vi "BonOMM-SAOMM.Test.vi"() -> ()   [LabVIEW 2011] (continued)
                                n1894 = local read "CmdPending"() -> (w5588:bool)
                                n1895 = case shown="True" w5588 {
                                tunnel: w5589 -> [_ w5595]
                                frame False {
                                }
                                frame True {
                                n1896 = local write "Error Code"(w5595) -> ()
                                }
                                }
                                n1897 = local read "FIFO d'erreur"() -> (w5591:T7)
                                n1898 = Bundle("ETCS", w5589, w5589, "ATTENTION!!\nLa commande STOP a échoué.\nVérifiez TCS.") -> (w5592:cluster{string, i32, i32, string})  [unwired: 1 in]
                                n1899 = Build Array (concatenate)(w5591, w5592) -> (w5590:T7)
                                n1900 = local write "FIFO d'erreur"(w5590) -> ()
                                }
                                frame True {
                                }
                                }
                                }
                                }
                                }
                                }
                                }
                                }
                              }
                              frame #2 {
                                w5598 = 0
                                w5599 = 0
                                w5596 = FALSE
                                # "Voir le fonctionnement de \"CMDPENDING\""
                                n1901 = property on="ModifDome" class="Bool (strict)"("Disabled"=w5599) -> ()  [unwired: 2 in, 2 out]
                                n1902 = property on="Écran" class="Bool (strict)"("Disabled"=w5599) -> ()  [unwired: 2 in, 2 out]
                                n1903 = property on="Range" class="Bool (strict)"("Disabled"=w5599) -> ()  [unwired: 2 in, 2 out]
                                n1904 = property on="Zénith" class="Bool (strict)"("Disabled"=w5599) -> ()  [unwired: 2 in, 2 out]
                                n1905 = property on="Synctel" class="Bool (strict)"("Disabled"=w5599) -> ()  [unwired: 2 in, 2 out]
                                n1906 = property on="Offset OK" class="Bool (strict)"("Disabled"=w5599) -> ()  [unwired: 2 in, 2 out]
                                n1907 = local read "CmdPending"() -> (w5597:bool)
                                n1908 = property on="GO" class="Bool (strict)"("Disabled"=w5598) -> ()  [unwired: 2 in, 2 out]
                                n1909 = property on="ModCoor" class="Bool (strict)"("Disabled"=w5598) -> ()  [unwired: 2 in, 2 out]
                                n1910 = property on="ModifFoyer" class="Bool (strict)"("Disabled"=w5598) -> ()  [unwired: 2 in, 2 out]
                                n1911 = property on="Coupole-Tél" class="Bool (strict)"("Disabled"=w5598) -> ()  [unwired: 2 in, 2 out]
                                n1912 = case shown="True" w5597 {
                                frame False {
                                }
                                frame True {
                                n1913 = local write "CmdPending"(FALSE) -> ()
                                }
                                }
                                n1914 = local write "ModifRotation"(w5596) -> ()
                                n1915 = property on="ModifRotation" class="Bool (strict)"("Blinking"=w5596) -> ()  [unwired: 2 in, 2 out]
                              }
                            }
                          }
                        }
                      }
                    }
                    n1916 = control-ref of="TERMINAL"() -> (w5495:refnum<vi>)
                    n1917 = control-ref of="Indicateur d'état"() -> (w5494:refnum<vi>)
                    n1918 = call "TERMINAL.vi"("Indicateur Refnum"=w5494, "Terminal Refnum"=w5495, "Indicateur d'état"="Modification de la rotation de la bonnette") -> ()
                  }
                }
              }
              event "ModifFoyer": Value Change {
                n1919 = event-data() -> ()  [unwired: 1 in, 5 out]
                n1920 = case shown="True" "ModifFoyer" {
                  frame False {
                  }
                  frame True {
                    n1921 = local read "Foyer"() -> (w5602:dbl)
                    n1922 = call "Set foyer.vi"("Foyer In"=w5602) -> ("Foyer Out"=w5604:dbl, "DONE"=w5605:bool, "sortie foyer sonde"=w5603:bool)  [unwired: 1 in]
                    n1923 = case shown="True" w5605 {
                      selector: w5605 -> [w5606 _]
                      tunnel: w5604 -> [_ w5610]
                      tunnel: w5603 -> [_ w5609]
                      tunnel: w5602 -> [_ w5608]
                      frame False {
                        n1924 = local write "ModifFoyer"(w5606) -> ()
                      }
                      frame True {
                        n1925 = Bundle By Name(cluster=T22 {"newFoyer"=0.0, "updSonde"=TRUE, "oldFoyer"=0.0}, "newFoyer"=w5610, "updSonde"=w5609, "oldFoyer"=w5608) -> (w5607:T22)
                        n1926 = call "EnqueueEvents.vi"("data"=w5607, "message"="Foyer.Ajuster") -> ()  [unwired: 1 in]
                      }
                    }
                  }
                }
              }
              event "ModifDome": Value Change {
                n1927 = event-data() -> ("NewVal"=w5613:bool)  [unwired: 1 in, 4 out]
                n1928 = case shown="True" w5613 {
                  frame False {
                  }
                  frame True {
                    n1929 = local read "Coupole"() -> (w5614:dbl)
                    n1930 = Number To Decimal String(number=w5614) -> (decimal integer string=w5615:string)  [unwired: 1 in]
                    n1931 = call "Set dome.vi"("Dome In"=w5614) -> ("DONE"=w5621:bool, "Dome Out"=w5620:dbl)
                    n1932 = Concatenate Strings("Synchronisation de la coupole sur " ("string"), w5615) -> (w5617:string)
                    n1933 = case shown="True" w5621 {
                      selector: w5621 -> [w5622 _]
                      tunnel: w5620 -> [_ w5623]
                      frame False {
                        n1934 = local write "ModifDome"(w5622) -> ()
                      }
                      frame True {
                        n1935 = stacked-sequence {
                          tunnel: w5623 -> [_ w5633 _]
                          frame #0 {
                            n1936 = control-ref of="TCS C actif"() -> (w5624:refnum<vi>)
                            n1937 = call "TCS-Wait4Flag.vi"("Raise Flag ?"=TRUE, "Ctl Refnum IN"=w5624) -> ()  [unwired: 8 in, 2 out]
                          }
                          frame #1 {
                            n1938 = control-ref of="TCS actif"() -> (w5626:refnum<vi>)
                            n1939 = local read "TCS VRN"() -> (w5632:refnum<visa-resource-name>)
                            n1940 = Build Array(w5633) -> (w5629:dbl[])
                            n1941 = call "EXCOM-CMD.vi"("VRN IN"=w5632, "Bool Refnum"=w5626, "Commande #"=2 ("NombredArguments"), "Args"=w5629) -> ("VRN OUT"=w5630:refnum<visa-resource-name>, "OK Done"=w5628:bool, "Error OUT"=w5627:errorcluster)  [unwired: 9 in]
                            n1942 = local write "TCS VRN"(w5630) -> ()
                            n1943 = local write "TCS Error"(w5627) -> ()
                            n1944 = case shown="False" w5628 {
                              selector: w5628 -> [w5634 w5638]
                              frame False {
                                n1945 = local write "ModifDome"(w5634) -> ()
                                n1946 = One Button Dialog(message="ATTENTION!!\nProblème d'ajustement\nde la position de la coupole.\nVérifiez TCS.", button name ("OK")="OK" ("nom du bouton (\"OK\")")) -> ()  [unwired: 1 out]
                              }
                              frame True {
                                n1947 = Not(x=w5638) -> (.not. x?=w5637:bool)
                                n1948 = local write "ModifDome"(w5637) -> ()
                              }
                            }
                          }
                          frame #2 {
                            n1949 = local write "TCS actif"(FALSE ("BONC-TCS")) -> ()
                          }
                        }
                      }
                    }
                    n1950 = control-ref of="TERMINAL"() -> (w5619:refnum<vi>)
                    n1951 = control-ref of="Indicateur d'état"() -> (w5618:refnum<vi>)
                    n1952 = call "TERMINAL.vi"("Indicateur Refnum"=w5618, "Terminal Refnum"=w5619, "Indicateur d'état"=w5617) -> ()
                  }
                }
              }
              event "Coupole-Tél": Value Change {
                n1953 = event-data() -> ()  [unwired: 1 in, 5 out]
                n1954 = Select(t="ON" ("string"), s="Coupole-Tél", f="OFF" ("string")) -> (s? t:f=w5649:string)
                n1955 = control-ref of="TERMINAL"() -> (w5653:refnum<vi>)
                n1956 = control-ref of="Indicateur d'état"() -> (w5652:refnum<vi>)
                n1957 = Concatenate Strings("AUTO DOME : " ("string"), w5649) -> (w5650:string)
                n1958 = call "TERMINAL.vi"("Indicateur Refnum"=w5652, "Terminal Refnum"=w5653, "Indicateur d'état"=w5650) -> ()
                n1959 = Boolean To (0,1)(Boolean="Coupole-Tél") -> (0, 1=w5655:i16)
                n1960 = To Double Precision Float(number=w5655) -> (double precision float=w5645:dbl)
                n1961 = Build Array(w5645) -> (w5644:dbl[])
                n1962 = control-ref of="TCS actif"() -> (w5640:refnum<vi>)
                n1963 = local read "TCS VRN"() -> (w5654:refnum<visa-resource-name>)
                n1964 = call "EXCOM-CMD.vi"("VRN IN"=w5654, "Bool Refnum"=w5640, "Commande #"=20 ("NombredArguments"), "Args"=w5644) -> ("VRN OUT"=w5643:refnum<visa-resource-name>, "OK Done"=w5641:bool, "Error OUT"=w5642:errorcluster)  [unwired: 9 in]
                n1965 = local write "TCS Error"(w5642) -> ()
                n1966 = local write "TCS VRN"(w5643) -> ()
                n1967 = case shown="False" w5641 {
                  frame False {
                    n1968 = One Button Dialog(message="ATTENTION!!\nLa commande DOME ON/OFF a échoué.\nVérifiez TCS.", button name ("OK")="OK" ("nom du bouton (\"OK\")")) -> ()  [unwired: 1 out]
                  }
                  frame True {
                  }
                }
              }
              event "Offset OK": Value Change {
                n1969 = event-data() -> ("NewVal"=w5659:bool)  [unwired: 1 in, 4 out]
                n1970 = case shown="True" w5659 {
                  frame False {
                  }
                  frame True {
                    # "OFFSET en\nsecondes d'arc"
                    # "Commande OFFSET\nSlew Enable"
                    # "MX"
                    # "MY"
                    # "Y"
                    # "X"
                    # "DEC"
                    # "AD"
                    n1971 = stacked-sequence {
                      seq-local: [_ w5704 _] -> [_ _ w5725]
                      tunnel: "Offset DEC" -> [w5668 w5702 _]
                      tunnel: "Offset RA" -> [w5671 w5703 _]
                      frame #0 {
                        n1972 = Number To Fractional String(number=w5668, precision (6)=i16 2) -> (F-format string=w5664:string)  [unwired: 2 in]
                        n1973 = Number To Fractional String(number=w5671, precision (6)=i16 2) -> (F-format string=w5666:string)  [unwired: 2 in]
                        n1974 = Concatenate Strings("Envoi manuel d'un offset de " ("string"), w5666, ", " ("string"), w5664) -> (w5663:string)
                        n1975 = local write "Offset OK"(FALSE) -> ()
                        n1976 = control-ref of="TERMINAL"() -> (w5672:refnum<vi>)
                        n1977 = control-ref of="Indicateur d'état"() -> (w5673:refnum<vi>)
                        n1978 = call "TERMINAL.vi"("Indicateur Refnum"=w5673, "Terminal Refnum"=w5672, "Indicateur d'état"=w5663) -> ()
                        "Offset en cours" <- TRUE ("Offset en cours")
                      }
                      frame #1 {
                        n1979 = control-ref of="MovingXY"() -> (w5676:refnum<vi>)
                        n1980 = control-ref of="SNR"() -> (w5677:refnum<vi>)
                        n1981 = control-ref of="TCS actif"() -> (w5697:refnum<vi>)
                        n1982 = control-ref of="Table actif"() -> (w5696:refnum<vi>)
                        n1983 = control-ref of="Position Z"() -> (w5695:refnum<vi>)
                        n1984 = control-ref of="StartServo"() -> (w5694:refnum<vi>)
                        n1985 = control-ref of="Mode"() -> (w5689:refnum<vi>)
                        n1986 = control-ref of="Servo"() -> (w5693:refnum<vi>)
                        n1987 = control-ref of="StopServo"() -> (w5692:refnum<vi>)
                        n1988 = control-ref of="DiffX"() -> (w5690:refnum<vi>)
                        n1989 = control-ref of="DiffY"() -> (w5691:refnum<vi>)
                        n1990 = local read "TableAstrom"() -> (w5686:T4)
                        n1991 = local read "FieldAstrom"() -> (w5688:T4)
                        n1992 = local read "GuiderAstrom"() -> (w5687:T4)
                        n1993 = local read "TCS VRN"() -> (w5685:refnum<visa-resource-name>)
                        n1994 = local read "TCS Error"() -> (w5684:errorcluster)
                        n1995 = local read "Table VRN"() -> (w5683:refnum<visa-resource-name>)
                        n1996 = local read "Table Error"() -> (w5682:errorcluster)
                        n1997 = Bundle("TableAstrom"=w5686, "FieldAstrom"=w5688, "GuiderAstrom"=w5687) -> (w5680:T40)  [unwired: 1 in]
                        n1998 = Bundle("TCS VRN"=w5685, "TCS Error"=w5684, "Table VRN"=w5683, "Table Error"=w5682) -> (w5679:T41)  [unwired: 1 in]
                        n1999 = Bundle("TCS actif"=w5697, "Table actif"=w5696, "Position Z"=w5695, "StartServo"=w5694, "Mode"=w5689, "Servo"=w5693, "StopServo"=w5692, "DiffX"=w5690, "DiffY"=w5691, "SNR"=w5677, "MovingXY"=w5676) -> (w5681:T42)  [unwired: 1 in]
                        n2000 = local read "OffsetAcc"() -> (w5678:dbl)
                        n2001 = while {
                          tunnel: [FALSE] -> w5675
                          stop <- w5707 continue-if-true
                          n2002 = local read "enfoncé"() -> (w5709:bool)
                          n2003 = Wait (ms)(milliseconds to wait=u32 200) -> ()  [unwired: 1 out]
                          n2004 = Not(x=w5709) -> (.not. x?=w5708:bool)
                          n2005 = local write "enfoncé"(w5708) -> ()
                          n2006 = local read "Offset en cours"() -> (w5707:bool)
                        }
                        n2007 = call "Cheesy_Offset.vi"("Communications_Cluster"=w5679, "Astrom_Cluster"=w5680, "RA offset"=w5703, "DEC offset"=w5702, "VariablesReferences"=w5681, "OffsetAccuracy (pixels)"=w5678) -> ("Error code"=w5701:u8, "Undo offset"=w5704:bool, "Warning code"=w5700:u8)  [unwired: 6 in, 1 out]
                        n2008 = To Unsigned Long Integer(number=w5700) -> (unsigned 32bit integer=w5698:u32)
                        n2009 = To Unsigned Long Integer(number=w5701) -> (unsigned 32bit integer=w5699:u32)
                        n2010 = flat-sequence {
                          tunnel: w5699 -> [w5713]
                          tunnel: w5698 -> [w5712]
                          frame #0 {
                            w5714 = u32 0 ("Error Code IN")
                            n2011 = local read "FIFO d'erreur"() -> (w5711:T7)
                            n2012 = call "Error_Format.vi"("FIFO IN"=w5711, "Error Code IN"=w5714, "Warning Code IN"=w5714, "Error Bit"=w5713, "Warning Bit"=w5712, "Source"="offset") -> ("FIFO OUT"=w5710:T7)  [unwired: 11 in, 2 out]
                            n2013 = local write "FIFO d'erreur"(w5710) -> ()
                          }
                          frame #1 {
                            n2014 = local write "Offset en cours"(FALSE ("Offset en cours")) -> ()
                          }
                        }
                        n2015 = local write "enfoncé"(w5675) -> ()
                      }
                      frame #2 {
                        w5726 = FALSE
                        # "Utile ?"
                        n2016 = local read "Table VRN"() -> (w5719:refnum<visa-resource-name>)
                        n2017 = local read "Table Error"() -> (w5718:errorcluster)
                        n2018 = control-ref of="Table actif"() -> (w5717:refnum<vi>)
                        n2019 = call "Newmark-Stop.vi"("Table VRN IN"=w5719, "Bool Refnum"=w5717, "Error IN"=w5718) -> ("Table VRN OUT"=w5721:refnum<visa-resource-name>, "Error OUT"=w5720:errorcluster)  [unwired: 11 in]
                        n2020 = local write "Table Error"(w5720) -> ()
                        n2021 = local write "Table VRN"(w5721) -> ()
                        n2022 = local write "RangeTable"(w5726) -> ()
                        n2023 = local write "Calibration"(w5726) -> ()
                        n2024 = local write "stoptable"(w5726) -> ()
                        n2025 = local write "Alacible"(w5726) -> ()
                        n2026 = local write "Origine"(w5726) -> ()
                        n2027 = local write "Centre"(w5726) -> ()
                        n2028 = case shown="False" w5725 {
                          tunnel: [" : réussi" " : échoué"] -> w5723
                          frame False {
                          }
                          frame True {
                          }
                        }
                        n2029 = local read "TERMINAL"() -> (w5724:string)
                        n2030 = Concatenate Strings(w5724, w5723) -> (w5722:string)
                        n2031 = local write "TERMINAL"(w5722) -> ()
                      }
                    }
                  }
                }
              }
              event "ChoixFiltre": Value Change {
                n2032 = event-data() -> ()  [unwired: 1 in, 5 out]
                n2033 = local read "MC-BonOMM VRN"() -> (w5729:refnum<visa-resource-name>)
                n2034 = stacked-sequence {
                  seq-local: [w5737 _ _ _] -> [_ w5800 _ _]
                  seq-local: [w5745 _ _ _] -> [_ w5797 _ _]
                  tunnel: w5729 -> [_ w5799 _ w5846]
                  frame #0 {
                    w5749 = 2
                    n2035 = local read "F#"() -> (w5735:i32)
                    n2036 = Number To Decimal String(number=w5735) -> (decimal integer string=w5736:string)  [unwired: 1 in]
                    n2037 = control-ref of="TERMINAL"() -> (w5741:refnum<vi>)
                    n2038 = control-ref of="Indicateur d'état"() -> (w5742:refnum<vi>)
                    n2039 = Unbundle("ChoixFiltre") -> ("filtre #1"=w5752:bool, "filtre #2"=w5753:bool, "filtre #3"=w5754:bool, "filtre #4"=w5755:bool, "filtre #5"=w5756:bool, "filtre #6"=w5757:bool)
                    n2040 = Build Array(w5752, w5753, w5754, w5755, w5756, w5757) -> (w5758:bool[])
                    n2041 = Search 1D Array(1D array=w5758, element=TRUE) -> (index of element=w5743:i32)  [unwired: 1 in]
                    n2042 = Increment(x=w5743) -> (x+1=w5737:i32)
                    n2043 = Number To Decimal String(number=w5737) -> (decimal integer string=w5738:string)  [unwired: 1 in]
                    n2044 = Concatenate Strings("Passage du filtre #", w5736, " au filtre #", w5738) -> (w5734:string)
                    n2045 = call "TERMINAL.vi"("Indicateur Refnum"=w5742, "Terminal Refnum"=w5741, "Indicateur d'état"=w5734) -> ()
                    n2046 = Not Equal To 0?(x=w5737) -> (x != 0?=w5744:bool)
                    n2047 = property on="ChoixFiltre" class="Clust (strict)"() -> ("Controls[]"=w5748:refnum<vi>[])  [unwired: 2 in, 2 out]
                    n2048 = case shown="True" w5744 {
                      selector: w5744 -> [w5782 _]
                      tunnel: w5743 -> [_ w5785]
                      tunnel: [w5782 w5784] -> w5745
                      frame False {
                      }
                      frame True {
                        n2049 = local read "Bypass Tech"() -> (w5783:bool)
                        n2050 = case shown="True" w5783 {
                          selector: w5783 -> [_ w5795]
                          tunnel: w5785 -> [w5793 _]
                          tunnel: [w5786 w5795] -> w5784
                          frame False {
                            n2051 = local read "Tableau des filtres"() -> (w5794:string[])
                            n2052 = Index Array(array=w5794, index=w5793) -> (element=w5792:string)
                            n2053 = Concatenate Strings("Désirez-vous passer au filtre " ("message"), w5792, " ?" ("message")) -> (w5789:string)
                            n2054 = Two Button Dialog(message=w5789, 1:"NON" ("F button name (\"Cancel\")"), 2:"OUI" ("T button name (\"OK\")")) -> (T button?=w5786:bool)
                          }
                          frame True {
                          }
                        }
                      }
                    }
                    n2055 = Index Array(array=w5748, index=w5743) -> (element=w5747:refnum<vi>)
                    n2056 = property class="Ctl"(reference=w5747, "Blinking"=TRUE) -> ()  [unwired: 1 in, 2 out]
                    n2057 = Index Array(array=w5748, index #1=0 ("indice"), index #2=1 ("indice"), index #3=2 ("indice"), index #4=3 ("indice"), index #5=4 ("indice"), index #6=5 ("indice")) -> (element #1=w5760:refnum<vi>, element #2=w5761:refnum<vi>, element #3=w5762:refnum<vi>, element #4=w5763:refnum<vi>, element #5=w5764:refnum<vi>, element #6=w5765:refnum<vi>)
                    n2058 = property class="Ctl"(reference=w5760, "Disabled"=w5749) -> ()  [unwired: 1 in, 2 out]
                    n2059 = property class="Ctl"(reference=w5761, "Disabled"=w5749) -> ()  [unwired: 1 in, 2 out]
                    n2060 = property class="Ctl"(reference=w5762, "Disabled"=w5749) -> ()  [unwired: 1 in, 2 out]
                    n2061 = property class="Ctl"(reference=w5763, "Disabled"=w5749) -> ()  [unwired: 1 in, 2 out]
                    n2062 = property class="Ctl"(reference=w5764, "Disabled"=w5749) -> ()  [unwired: 1 in, 2 out]
                    n2063 = property class="Ctl"(reference=w5765, "Disabled"=w5749) -> ()  [unwired: 1 in, 2 out]
                    n2064 = local read "Tableau des filtres"() -> (w5733:string[])
                    n2065 = Current VI's Menubar() -> (w5730:refnum<k9>)
                    n2066 = for {
                      tunnel: w5733 -> [w5774] mode=indexing
                      tunnel: "@@" -> [w5778]
                      tunnel: "raf_" -> [w5779]
                      tunnel: w5730 -> [w5775]
                      tunnel: [w5773] -> _ mode=indexing
                      i -> [w5780]
                      n2067 = Number To Decimal String(number=w5780, width (-)=i16 1) -> (decimal integer string=w5777:string)
                      n2068 = Concatenate Strings(w5779, w5774, w5778, w5777) -> (w5776:string)
                      n2069 = Set Menu Item Info(6:FALSE ("checked"), 7:w5776, 9:TRUE ("enabled"), 10:w5774, 11:w5775) -> (0:w5773:errorcluster)  [unwired: 2 in, 1 out]
                    }
                  }
                  frame #1 {
                    n2070 = Not Equal To 0?(x=w5800) -> (x != 0?=w5798:bool)
                    n2071 = And(x=w5798, y=w5797) -> (x .and. y?=w5796:bool)
                    n2072 = case shown="True" w5796 {
                      tunnel: w5800 -> [_ w5801]
                      tunnel: w5799 -> [_ w5802]
                      frame False {
                      }
                      frame True {
                        n2073 = Number To Decimal String(number=w5801, width (-)=i16 1) -> (decimal integer string=w5803:string)
                        n2074 = VISA Write(VISA resource name=w5802, write buffer=w5803) -> (VISA resource name out=w5804:refnum<visa-resource-name>)  [unwired: 1 in, 2 out]
                        n2075 = while {
                          tunnel: w5804 -> [w5814]
                          tunnel: w5801 -> [w5813]
                          stop <- w5812 stop-if-true
                          n2076 = while {
                            tunnel: w5814 -> [w5825]
                            tunnel: [w5824] -> w5809
                            tunnel: [w5823] -> w5807
                            i -> [w5828]
                            stop <- w5821 stop-if-true
                            n2077 = local read "Annulation en cours"() -> (w5820:bool)
                            n2078 = property class="Instr"(reference=w5825) -> (reference out=w5824:refnum<visa-resource-name>, "Serial Settings:Number of Bytes at Serial Port"=w5829:u32)  [unwired: 1 in, 1 out]
                            n2079 = Not Equal To 0?(x=w5829) -> (x != 0?=w5823:bool)
                            n2080 = call "Max-iteration.vi"("i max"=100, "i act"=w5828, "Valeur entrante"=w5823) -> ("break ?"=w5822:bool)
                            n2081 = Or(x=w5820, y=w5822) -> (x .or. y?=w5821:bool)
                            n2082 = Wait Until Next ms Multiple(millisecond multiple=u32 100) -> ()  [unwired: 1 out]
                          }
                          n2083 = case shown="True" w5807 {
                            tunnel: w5809 -> [_ w5819]
                            tunnel: [0 w5816] -> w5808
                            frame False {
                            }
                            frame True {
                              n2084 = VISA Read(VISA resource name=w5819, byte count=u32 1) -> (read buffer=w5817:string)  [unwired: 1 in, 3 out]
                              n2085 = Decimal String To Number(string=w5817) -> (number=w5816:i32)  [unwired: 2 in, 1 out]
                            }
                          }
                          n2086 = Not(x=w5807) -> (.not. x?=w5811:bool)
                          n2087 = local write "F#"(w5808) -> ()
                          n2088 = Equal?(x=w5808, y=w5813) -> (x = y?=w5806:bool)
                          n2089 = local read "Annulation en cours"() -> (w5810:bool)
                          n2090 = Compound Arithmetic op=OR(w5806, w5811, w5810) -> (w5812:bool)
                        }
                      }
                    }
                  }
                  frame #2 {
                    n2091 = local read "Annulation en cours"() -> (w5830:bool)
                    n2092 = case shown="False" w5830 {
                      frame False {
                        n2093 = local read "MC_connect"() -> (w5831:bool)
                        n2094 = Wait (ms)(milliseconds to wait=u32 500) -> ()  [unwired: 1 out]
                        n2095 = case shown="False" w5831 {
                          frame False {
                            n2096 = One Button Dialog(message="Errreur lors du déplacement de la roue") -> ()  [unwired: 1 in, 1 out]
                          }
                          frame True {
                          }
                        }
                      }
                      frame True {
                      }
                    }
                  }
                  frame #3 {
                    w5837 = u8 0 ("byte count")
                    w5847 = FALSE
                    n2097 = local read "Annulation en cours"() -> (w5834:bool)
                    n2098 = case shown="False" w5834 {
                      tunnel: w5846 -> [w5869 _]
                      frame False {
                        n2099 = call "MC-BonOMM_talker.vi"("MC-BonOMM VRN"=w5869, "Commande"="q" ("write buffer"), "byte count"=u32 1, "Timeout (ms)"=1000, "answer=command?"=FALSE) -> ("Answer"=w5864:string, "ok ?"=w5863:bool)
                        n2100 = local write "MC_connect"(w5863) -> ()
                        n2101 = Decimal String To Number(string=w5864) -> (number=w5868:i32)  [unwired: 2 in, 1 out]
                        n2102 = local write "F#"(w5868) -> ()
                        n2103 = case shown="1..6" w5868 {
                          selector: w5868 -> [w5879 _]
                          frame 1..6 {
                            w5870 = TRUE ("enabled")
                            n2104 = Decrement(x=w5879) -> (x-1=w5871:i32)
                            n2105 = local read "Tableau des filtres"() -> (w5880:string[])
                            n2106 = Index Array(array=w5880, index=w5871) -> (element=w5872:string)
                            n2107 = Number To Decimal String(number=w5871, width (-)=i16 1) -> (decimal integer string=w5876:string)
                            n2108 = local write "filtre_nom"(w5872) -> ()
                            n2109 = Concatenate Strings("raf_", w5872, "@@", w5876) -> (w5878:string)
                            n2110 = Current VI's Menubar() -> (w5877:refnum<k9>)
                            n2111 = Set Menu Item Info(6:w5870, 7:w5878, 9:w5870, 10:w5872, 11:w5877) -> ()  [unwired: 2 in, 2 out]
                          }
                          frame 0, Default {
                            n2112 = local write "filtre_nom"("") -> ()
                          }
                        }
                      }
                      frame True {
                        n2113 = local read "MC-BonOMM VRN"() -> (w5883:refnum<visa-resource-name>)
                        n2114 = local read "Périphérique"() -> (w5887:u16)
                        n2115 = VISA Write(VISA resource name=w5883, write buffer="r") -> (VISA resource name out=w5884:refnum<visa-resource-name>)  [unwired: 1 in, 2 out]
                        n2116 = Equal To 0?(x=w5887) -> (x = 0?=w5888:bool)
                        n2117 = Select(t="f", s=w5888, f="o") -> (s? t:f=w5891:string)
                        n2118 = flat-sequence {
                          tunnel: w5884 -> [w5913]
                          tunnel: [w5913] -> w5894
                          frame #0 {
                            n2119 = Wait (ms)(milliseconds to wait=u32 2000) -> ()  [unwired: 1 out]
                          }
                        }
                        n2120 = call "MC-BonOMM_talker.vi"("MC-BonOMM VRN"=w5894, "Commande"=w5891, "byte count"=u32 1, "Timeout (ms)"=2000, "answer=command?"=TRUE) -> ("ok ?"=w5882:bool)  [unwired: 1 out]
                        n2121 = local write "MC_connect"(w5882) -> ()
                        n2122 = case shown="True" w5882 {
                          tunnel: w5894 -> [_ w5896]
                          frame False {
                            n2123 = One Button Dialog(message="Erreur lors de l'arrêt, essayez \"reconnecter\"") -> ()  [unwired: 1 in, 1 out]
                          }
                          frame True {
                            n2124 = flat-sequence {
                              tunnel: [w5906] -> w5897
                              tunnel: w5896 -> [w5905]
                              frame #0 {
                                n2125 = Wait (ms)(milliseconds to wait=u32 500) -> ()  [unwired: 1 out]
                              }
                              frame #1 {
                                n2126 = call "MC-BonOMM_talker.vi"("MC-BonOMM VRN"=w5905, "Commande"="q", "byte count"=u32 1, "Timeout (ms)"=8000, "answer=command?"=FALSE) -> ("Answer"=w5901:string, "ok ?"=w5900:bool)
                                n2127 = local write "MC_connect"(w5900) -> ()
                                n2128 = Decimal String To Number(string=w5901) -> (number=w5906:i32)  [unwired: 2 in, 1 out]
                              }
                            }
                            n2129 = local write "F#"(w5897) -> ()
                            n2130 = case shown="1..6" w5897 {
                              selector: w5897 -> [w5907 _]
                              frame 1..6 {
                                n2131 = Decrement(x=w5907) -> (x-1=w5910:i32)
                                n2132 = local read "Tableau des filtres"() -> (w5908:string[])
                                n2133 = Index Array(array=w5908, index=w5910) -> (element=w5909:string)
                                n2134 = local write "filtre_nom"(w5909) -> ()
                              }
                              frame 0, Default {
                                n2135 = local write "filtre_nom"("") -> ()
                              }
                            }
                          }
                        }
                      }
                    }
                    n2136 = property on="ChoixFiltre" class="Clust (strict)"() -> ("Controls[]"=w5848:refnum<vi>[])  [unwired: 2 in, 2 out]
                    n2137 = Index Array(array=w5848, index #1=0 ("indice"), index #2=1 ("indice"), index #3=2 ("indice"), index #4=3 ("indice"), index #5=4 ("indice"), index #6=5 ("indice")) -> (element #1=w5850:refnum<vi>, element #2=w5851:refnum<vi>, element #3=w5852:refnum<vi>, element #4=w5853:refnum<vi>, element #5=w5854:refnum<vi>, element #6=w5855:refnum<vi>)
                    n2138 = property class="Ctl"(reference=w5850, "Blinking"=w5847) -> (reference out=w5845:refnum<vi>)  [unwired: 1 in, 1 out]
                    n2139 = property class="Ctl"(reference=w5851, "Blinking"=w5847) -> (reference out=w5844:refnum<vi>)  [unwired: 1 in, 1 out]
                    n2140 = property class="Ctl"(reference=w5852, "Blinking"=w5847) -> (reference out=w5843:refnum<vi>)  [unwired: 1 in, 1 out]
                    n2141 = property class="Ctl"(reference=w5853, "Blinking"=w5847) -> (reference out=w5842:refnum<vi>)  [unwired: 1 in, 1 out]
                    n2142 = property class="Ctl"(reference=w5854, "Blinking"=w5847) -> (reference out=w5841:refnum<vi>)  [unwired: 1 in, 1 out]
                    n2143 = property class="Ctl"(reference=w5855, "Blinking"=w5847) -> (reference out=w5840:refnum<vi>)  [unwired: 1 in, 1 out]
                    n2144 = Bundle(w5847, w5847, w5847, w5847, w5847, w5847) -> (w5861:cluster{bool, bool, bool, bool, bool, bool})  [unwired: 1 in]
                    n2145 = local read "Périphérique"() -> (w5839:u16)
                    n2146 = property class="Ctl"(reference=w5845, "Disabled"=w5837) -> ()  [unwired: 1 in, 2 out]
                    n2147 = property class="Ctl"(reference=w5844, "Disabled"=w5837) -> ()  [unwired: 1 in, 2 out]
                    n2148 = property class="Ctl"(reference=w5843, "Disabled"=w5837) -> ()  [unwired: 1 in, 2 out]
                    n2149 = property class="Ctl"(reference=w5842, "Disabled"=w5837) -> ()  [unwired: 1 in, 2 out]
                    n2150 = property class="Ctl"(reference=w5841, "Disabled"=w5837) -> ()  [unwired: 1 in, 2 out]
                    n2151 = property on="ChoixFiltre" class="Clust (strict)"("Value"=w5861) -> ()  [unwired: 2 in, 2 out]
                    n2152 = Equal To 0?(x=w5839) -> (x = 0?=w5838:bool)
                    n2153 = Select(t=w5837, s=w5838, f=u8 2) -> (s? t:f=w5835:u8)
                    n2154 = property class="Ctl"(reference=w5840, "Disabled"=w5835) -> ()  [unwired: 1 in, 2 out]
                  }
                }
              }
              event "Périphérique", "reconnect": Value Change {
                n2155 = event-data() -> ()  [unwired: 1 in, 5 out]
                n2156 = Equal?(x="Périphérique", y=u16 3) -> (x = y?=w5934:bool)
                n2157 = Equal?(x="Périphérique", y=u16 4) -> (x = y?=w5937:bool)
                n2158 = property on="AngOK" class="Bool"("Visible"=w5937) -> ()  [unwired: 2 in, 2 out]
                n2159 = property on="PAS" class="DigNum (strict)"("Visible"=w5937) -> ()  [unwired: 2 in, 2 out]
                n2160 = property on="ANG+" class="Bool"("Visible"=w5937) -> ()  [unwired: 2 in, 2 out]
                n2161 = property on="Set angle" class="DigNum (strict)"("Visible"=w5937) -> ()  [unwired: 2 in, 2 out]
                n2162 = property on="ANG-" class="Bool"("Visible"=w5937) -> ()  [unwired: 2 in, 2 out]
                n2163 = property on="Arc" class="Bool (strict)"("Visible"=w5934) -> ()  [unwired: 2 in, 2 out]
                n2164 = property on="Flat" class="Bool (strict)"("Visible"=w5934) -> ()  [unwired: 2 in, 2 out]
                n2165 = property on="Néon" class="Bool (strict)"("Visible"=w5934) -> ()  [unwired: 2 in, 2 out]
                n2166 = Equal?(x="Périphérique", y=u16 2) -> (x = y?=w5925:bool)
                n2167 = local write "reconnect"(FALSE ("reconnect")) -> ()
                n2168 = property on="SET ZERO" class="Bool"("Visible"=w5925) -> ()  [unwired: 2 in, 2 out]
                n2169 = property on="ST+" class="Bool (strict)"("Visible"=w5925) -> ()  [unwired: 2 in, 2 out]
                n2170 = property on="ST-" class="Bool (strict)"("Visible"=w5925) -> ()  [unwired: 2 in, 2 out]
                n2171 = property on="ST_RAZ" class="Bool"("Visible"=w5925) -> ()  [unwired: 2 in, 2 out]
                n2172 = property on="ST_SPD" class="Slide (strict)"("Visible"=w5925) -> ()  [unwired: 2 in, 2 out]
                n2173 = Equal?(x="Périphérique", y=u16 0) -> (x = y?=w5927:bool)
                n2174 = Equal?(x="Périphérique", y=u16 1) -> (x = y?=w5926:bool)
                n2175 = Or(x=w5927, y=w5926) -> (x .or. y?=w5915:bool)
                n2176 = Select(t=u8 0 ("y"), s=w5927, f=u8 2 ("y")) -> (s? t:f=w5930:u8)
                n2177 = property on="filtre #6" class="Bool (strict)"("Disabled"=w5930) -> ()  [unwired: 2 in, 2 out]
                n2178 = Build Array(w5927, w5926, w5925) -> (w5924:bool[])
                n2179 = Or(x=w5915, y=w5925) -> (x .or. y?=w5916:bool)
                n2180 = property on="reconnect" class="Bool (strict)"("Visible"=w5916) -> ()  [unwired: 2 in, 2 out]
                n2181 = Boolean Array To Number(Boolean array=w5924) -> (number=w5923:u32)
                n2182 = property on="ChoixFiltre" class="Clust (strict)"("Visible"=w5915) -> ()  [unwired: 2 in, 2 out]
                n2183 = property on="filtre_nom" class="Str"("Visible"=w5915) -> ()  [unwired: 2 in, 2 out]
                n2184 = property on="q-raf" class="Bool (strict)"("Visible"=w5915) -> ()  [unwired: 2 in, 2 out]
                n2185 = property on="cancel-raf" class="Bool (strict)"("Visible"=w5915) -> ()  [unwired: 2 in, 2 out]
                n2186 = property on="change_filtre_liste" class="Bool (strict)"("Visible"=w5915) -> ()  [unwired: 2 in, 2 out]
                n2187 = property on="F#" class="DigNum (strict)"("Visible"=w5915) -> ()  [unwired: 2 in, 2 out]
                n2188 = case shown="True" w5916 {
                  tunnel: w5923 -> [_ w5940]
                  frame False {
                  }
                  frame True {
                    n2189 = flat-sequence {
                      tunnel: w5940 -> [w5944]
                      tunnel: [w5944] -> w5939
                      tunnel: w5939 -> [w5964]
                      frame #0 {
                        n2190 = flat-sequence {
                          tunnel: w5941 -> [w5948]
                          frame #0 {
                            n2191 = Wait (ms)(milliseconds to wait=u32 2000) -> ()  [unwired: 1 out]
                          }
                          frame #1 {
                            n2192 = property class="Instr"(reference=w5948) -> (reference out=w5947:refnum<visa-resource-name>, "Serial Settings:Number of Bytes at Serial Port"=w5946:u32)  [unwired: 1 in, 1 out]
                            n2193 = local write "MC_connect"(FALSE ("MC_connect")) -> ()
                            n2194 = VISA Read(VISA resource name=w5947, byte count=w5946) -> ()  [unwired: 1 in, 4 out]
                          }
                        }
                        n2195 = local read "MC-BonOMM VRN"() -> (w5943:refnum<visa-resource-name>)
                        n2196 = VISA Write(VISA resource name=w5943, write buffer="r" ("Commande")) -> (VISA resource name out=w5941:refnum<visa-resource-name>)  [unwired: 1 in, 2 out]
                      }
                      frame #1 {
                        n2197 = local read "MC-BonOMM VRN"() -> (w5960:refnum<visa-resource-name>)
                        n2198 = call "MC-BonOMM_talker.vi"("MC-BonOMM VRN"=w5960, "Commande"="m", "byte count"=u32 1, "Timeout (ms)"=2000, "answer=command?"=FALSE) -> ("Answer"=w5954:string, "ok ?"=w5957:bool)
                        n2199 = Equal?(x="f", y=w5954) -> (x = y?=w5953:bool)
                        n2200 = Equal?(x=w5954, y="x") -> (x = y?=w5952:bool)
                        n2201 = Or(x=w5953, y=w5952) -> (x .or. y?=w5951:bool)
                        n2202 = And(x=w5951, y=w5957) -> (x .and. y?=w5958:bool)
                        n2203 = case shown="True" w5958 {
                          tunnel: w5964 -> [_ w5970]
                          tunnel: [w5965 w5969] -> w5950
                          frame False {
                            n2204 = One Button Dialog(message="Problème de communication avec MC-BonOMM", button name ("OK")="Oups :(") -> (true=w5966:bool)
                            n2205 = Not(x=w5966) -> (.not. x?=w5965:bool)
                          }
                          frame True {
                            n2206 = stacked-sequence {
                              tunnel: w5970 -> [w5975 w6001]
                              tunnel: [_ w5999] -> w5969
                              frame #0 {
                                n2207 = local read "MC-BonOMM VRN"() -> (w5977:refnum<visa-resource-name>)
                                n2208 = case shown="1, Default" w5975 {
                                tunnel: ["f" "o" "x"] -> w5974
                                frame 1, Default {
                                }
                                frame 2 {
                                }
                                frame 4 {
                                }
                                }
                                n2209 = call "MC-BonOMM_talker.vi"("MC-BonOMM VRN"=w5977, "Commande"=w5974, "Timeout (ms)"=2000, "answer=command?"=TRUE) -> ("ok ?"=w5971:bool)  [unwired: 1 in, 1 out]
                                n2210 = local write "MC_connect"(w5971) -> ()
                                n2211 = Equal?(x=w5974, y="f") -> (x = y?=w5972:bool)
                                n2212 = case shown="False" w5971 {
                                frame False {
                                n2213 = One Button Dialog(message="Erreur lors du changement de mode ...") -> ()  [unwired: 1 in, 1 out]
                                }
                                frame True {
                                }
                                }
                                n2214 = case shown="True" w5972 {
                                tunnel: w5971 -> [_ w5979]
                                frame False {
                                }
                                frame True {
                                n2215 = local read "Tableau des filtres"() -> (w5983:string[])
                                n2216 = Current VI's Menubar() -> (w5980:refnum<k9>)
                                n2217 = for {
                                tunnel: w5983 -> [w5986] mode=indexing
                                tunnel: "@@" -> [w5991]
                                tunnel: "raf_" -> [w5992]
                                tunnel: w5980 -> [w5988]
                                tunnel: w5979 -> [w5987]
                                tunnel: [w5985] -> _ mode=indexing
                                i -> [w5993]
                                n2218 = Number To Decimal String(number=w5993, width (-)=i16 1) -> (decimal integer string=w5990:string)
                                n2219 = Concatenate Strings(w5992, w5986, w5991, w5990) -> (w5989:string)
                                n2220 = Set Menu Item Info(6:FALSE ("checked"), 7:w5989, 9:w5987, 10:w5986, 11:w5988) -> (0:w5985:errorcluster)  [unwired: 2 in, 1 out]
                                }
                                }
                                }
                              }
                              frame #1 {
                                n2221 = local read "MC-BonOMM VRN"() -> (w6000:refnum<visa-resource-name>)
                                n2222 = case shown="1, 2, Default" w6001 {
                                tunnel: w6000 -> [w6007 w6023]
                                tunnel: [w6005 w6022] -> w5999
                                frame 1, 2, Default {
                                n2223 = call "MC-BonOMM_talker.vi"("MC-BonOMM VRN"=w6007, "Commande"="q", "byte count"=u32 1, "Timeout (ms)"=8000, "answer=command?"=FALSE) -> ("Answer"=w6006:string, "ok ?"=w6005:bool)
                                n2224 = Decimal String To Number(string=w6006) -> (number=w6009:i32)  [unwired: 2 in, 1 out]
                                n2225 = local write "F#"(w6009) -> ()
                                n2226 = case shown="1..6" w6009 {
                                selector: w6009 -> [w6019 _]
                                frame 1..6 {
                                n2227 = local read "Tableau des filtres"() -> (w6020:string[])
                                n2228 = Decrement(x=w6019) -> (x-1=w6015:i32)
                                n2229 = Index Array(array=w6020, index=w6015) -> (element=w6010:string)
                                n2230 = Number To Decimal String(number=w6015, width (-)=i16 1) -> (decimal integer string=w6014:string)
                                n2231 = Current VI's Menubar() -> (w6013:refnum<k9>)
                                n2232 = local write "filtre_nom"(w6010) -> ()
                                n2233 = Concatenate Strings("raf_", w6010, "@@", w6014) -> (w6012:string)
                                n2234 = Set Menu Item Info(6:TRUE ("enabled"), 7:w6012, 10:w6010, 11:w6013) -> ()  [unwired: 3 in, 2 out]
                                }
                                frame 0, Default {
                                n2235 = local write "filtre_nom"("") -> ()
                                }
                                }
                                }
                                frame 4 {
                                n2236 = local read "ST_SPD"() -> (w6024:dbl)
                                n2237 = call "Change_speed.vi"("ST_SPD"=w6024, "MC-BonOMM VRN"=w6023) -> ("Connected?"=w6022:bool)
                                n2238 = case shown="False" w6022 {
                                frame False {
                                n2239 = property on="Périphérique" class="Ring (strict)"("Value (Signaling)"=u16 3) -> ()  [unwired: 2 in, 2 out]
                                }
                                frame True {
                                }
                                }
                                }
                                }
                              }
                            }
                          }
                        }
                        "MC_connect" <- w5950
                      }
                    }
                  }
                }
                n2240 = property on="Périphérique" class="Ring (strict)"() -> ("Ring Text.Text"=w5917:string)  [unwired: 2 in, 2 out]
                n2241 = control-ref of="TERMINAL"() -> (w5922:refnum<vi>)
                n2242 = control-ref of="Indicateur d'état"() -> (w5921:refnum<vi>)
                n2243 = Concatenate Strings("Changement du périphérique pour \"", w5917, "\"") -> (w5918:string)
                n2244 = call "TERMINAL.vi"("Indicateur Refnum"=w5921, "Terminal Refnum"=w5922, "Indicateur d'état"=w5918) -> ()
              }
              event "change_filtre_liste": Value Change {
                n2245 = event-data() -> ()  [unwired: 1 in, 6 out]
                n2246 = case shown="True" "change_filtre_liste" {
                  frame False {
                  }
                  frame True {
                    n2247 = flat-sequence {
                      frame #0 {
                        n2248 = local read "Tableau des filtres"() -> (w6032:string[])
                        n2249 = Current VI's Menubar() -> (w6030:refnum<k9>)
                        n2250 = local write "change_filtre_liste"(FALSE) -> ()
                        n2251 = call "RaFMenuFixer.vi"("Tableau des filtres"=w6032, "Prefix"="raf_") -> ("Item Tags"=w6028:string[])  [unwired: 8 in, 1 out]
                        n2252 = call "ChoixFiltres.vi"("Ordre des filtres Avant"=w6032) -> ("Ordre des filtres Après"=w6034:string[])
                        n2253 = Delete Menu Items(7:w6028, 8:"main_Roue à filtres" ("menu tag"), 9:w6030) -> (0:w6027:errorcluster, 3:w6031:refnum<k9>)  [unwired: 1 in]
                        n2254 = local write "Tableau des filtres"(w6034) -> ()
                        n2255 = control-ref of="TERMINAL"() -> (w6044:refnum<vi>)
                        n2256 = control-ref of="Indicateur d'état"() -> (w6045:refnum<vi>)
                        n2257 = call "RaFMenuFixer.vi"("Tableau des filtres"=w6034, "Prefix"="raf_") -> ("Item Tags"=w6035:string[], "Item Names"=w6036:string[])  [unwired: 8 in]
                        n2258 = Insert Menu Items(5:"main_Roue à filtres" ("menu tag"), 6:w6027, 7:w6035, 8:w6036, 9:w6031) -> ()  [unwired: 1 in, 3 out]
                        n2259 = call "TERMINAL.vi"("Indicateur Refnum"=w6045, "Terminal Refnum"=w6044, "Indicateur d'état"="Modification de la liste des filtres") -> ()
                        n2260 = Array Size(array=w6034) -> (size(s)=w6039:i32)
                        n2261 = Array Subset(array=w6035, index=2, length=w6039) -> ()  [unwired: 1 out]
                        n2262 = Array Subset(array=w6036, index=2, length=w6039) -> ()  [unwired: 1 out]
                      }
                      frame #1 {
                        n2263 = property on="q-raf" class="Bool (strict)"("Val(Sgnl)"=TRUE ("Value (Signaling)")) -> ()  [unwired: 2 in, 2 out]
                      }
                    }
                  }
                }
              }
              event "q-raf": Value Change {
                n2264 = event-data() -> ()  [unwired: 1 in, 6 out]
                n2265 = case shown="True" "q-raf" {
                  frame False {
                  }
                  frame True {
                    n2266 = local read "MC-BonOMM VRN"() -> (w6052:refnum<visa-resource-name>)
                    n2267 = local write "q-raf"(FALSE) -> ()
                    n2268 = VISA Write(VISA resource name=w6052, write buffer="q") -> (VISA resource name out=w6053:refnum<visa-resource-name>)  [unwired: 1 in, 2 out]
                    n2269 = VISA Read(VISA resource name=w6053, byte count=u32 1) -> (read buffer=w6055:string)  [unwired: 1 in, 3 out]
                    n2270 = control-ref of="TERMINAL"() -> (w6049:refnum<vi>)
                    n2271 = control-ref of="Indicateur d'état"() -> (w6050:refnum<vi>)
                    n2272 = Decimal String To Number(string=w6055) -> (number=w6057:i32)  [unwired: 2 in, 1 out]
                    n2273 = call "TERMINAL.vi"("Indicateur Refnum"=w6050, "Terminal Refnum"=w6049, "Indicateur d'état"="Actualisation de la position de la roue à filtre") -> ()
                    n2274 = local write "F#"(w6057) -> ()
                    n2275 = case shown="1..6" w6057 {
                      selector: w6057 -> [w6069 _]
                      frame 1..6 {
                        n2276 = Decrement(x=w6069) -> (x-1=w6058:i32)
                        n2277 = local read "Tableau des filtres"() -> (w6070:string[])
                        n2278 = Index Array(array=w6070, index=w6058) -> (element=→"filtre_nom":string)
                        n2279 = local read "Tableau des filtres"() -> (w6068:string[])
                        n2280 = Index Array(array=w6068, index=w6058) -> (element=w6060:string)
                        n2281 = Number To Decimal String(number=w6058, width (-)=i16 1) -> (decimal integer string=w6064:string)
                        n2282 = Current VI's Menubar() -> (w6063:refnum<k9>)
                        n2283 = Concatenate Strings("raf_", w6060, "@@", w6064) -> (w6062:string)
                        n2284 = Set Menu Item Info(6:TRUE ("enabled"), 7:w6062, 10:w6060, 11:w6063) -> ()  [unwired: 3 in, 2 out]
                      }
                      frame 0, Default {
                        n2285 = local write "filtre_nom"("") -> ()
                      }
                    }
                  }
                }
              }
              event "AngOK": Value Change {
                n2286 = event-data() -> ("NewVal"=w6072:bool)  [unwired: 1 in, 4 out]
                n2287 = case shown="True" w6072 {
                  frame False {
                  }
                  frame True {
                    # "160000 pas/tour"
                    n2288 = Divide(x="Set angle", y=360.0) -> (x/y=w6075:dbl)
                    n2289 = Multiply(x=w6075, y=160000.0) -> (x*y=w6073:dbl)
                    n2290 = To Long Integer(number=w6073) -> ()  [unwired: 1 out]
                  }
                }
              }
              event "ANG+", "ANG-": Value Change {
                n2291 = event-data() -> ()  [unwired: 1 in, 5 out]
                n2292 = case shown="True" "ANG+" {
                  tunnel: "PAS" -> [_ _]
                  frame False {
                  }
                  frame True {
                  }
                }
              }
              event "Load_obj": Value Change {
                n2293 = event-data() -> ()  [unwired: 1 in, 5 out]
                n2294 = case shown="True" "Load_obj" {
                  frame False {
                  }
                  frame True {
                    n2295 = property on="Obslib" class="Tbl (strict)"() -> ("Selection Start"=w6084:T43)  [unwired: 2 in, 2 out]
                    n2296 = local read "Obslib"() -> (w6096:string[][])
                    n2297 = local write "Load_obj"(FALSE ("Charger le l'objet #1")) -> ()
                    n2298 = Unbundle(w6084) -> ("Row"=w6097:i32)  [unwired: 1 out]
                    n2299 = Index Array(array=w6096, index (row)=w6097) -> (element=w6081:string[])  [unwired: 1 in]
                    n2300 = Index Array(array=w6081, index #1=0, index #2=1, index #3=2) -> (element #1=w6093:string, element #2=w6094:string, element #3=w6095:string)
                    n2301 = Concatenate Strings("Désirez-vous charger la coordonnées : \nRA = ", w6093, "\nDEC = ", w6094, "\nEpoch = ", w6095) -> (w6088:string)
                    n2302 = Two Button Dialog(message=w6088, 1:"NON" ("F button name (\"Cancel\")"), 2:"OUI" ("T button name (\"OK\")")) -> (T button?=w6092:bool)
                    n2303 = case shown="True" w6092 {
                      tunnel: w6093 -> [_ w6104]
                      tunnel: w6094 -> [_ w6103]
                      tunnel: w6095 -> [_ w6102]
                      tunnel: w6081 -> [_ w6101]
                      tunnel: w6081 -> [_ w6099]
                      frame False {
                      }
                      frame True {
                        n2304 = flat-sequence {
                          tunnel: w6104 -> [w6125]
                          tunnel: w6103 -> [w6123]
                          tunnel: w6102 -> [w6122]
                          tunnel: w6101 -> [w6140]
                          tunnel: [w6131] -> w6100
                          tunnel: w6100 -> [w6147]
                          tunnel: w6099 -> [w6148]
                          frame #0 {
                            w6124 = ", "
                            w6129 = 3600.0 ("y")
                            n2305 = call "time-str-to-time-dbl-RA.vi"("Chaîne"=w6125) -> ("TCS_coords"=w6120:dbl)
                            n2306 = call "time-str-to-time-dbl-DEC.vi"("Chaîne"=w6123) -> ("TCS_coords"=w6119:dbl)
                            n2307 = call "time-str-to-time-dbl.vi"("Chaîne"=w6122) -> ("TCS_coords"=w6118:dbl)
                            n2308 = control-ref of="TERMINAL"() -> (w6128:refnum<vi>)
                            n2309 = control-ref of="Indicateur d'état"() -> (w6127:refnum<vi>)
                            n2310 = Multiply(x=w6120, y=w6129) -> (x*y=w6116:dbl)
                            n2311 = control-ref of="TCS actif"() -> (w6107:refnum<vi>)
                            n2312 = local read "TCS VRN"() -> (w6130:refnum<visa-resource-name>)
                            n2313 = local read "LST"() -> (w6110:dbl)
                            n2314 = Multiply(x=w6119, y=w6129) -> (x*y=w6117:dbl)
                            n2315 = Concatenate Strings("Chargement de l'objet : ", w6125, w6124, w6123, w6124, w6122) -> (w6121:string)
                            n2316 = Build Array(w6120, w6119, w6118) -> (w6105:dbl[])
                            n2317 = call "Object_properties.vi"("Target RA"=w6116, "Target DEC"=w6117, "Target Epoch"=w6118, "Sideral Time"=w6110) -> ("NO RA"=w6115:string, "NO DEC"=w6114:string, "NO Epoch"=w6113:dbl, "NO HA"=w6112:dbl, "NO AM"=w6111:dbl)  [unwired: 7 in]
                            n2318 = call "TERMINAL.vi"("Indicateur Refnum"=w6127, "Terminal Refnum"=w6128, "Indicateur d'état"=w6121) -> ()
                            n2319 = call "EXCOM-CMD.vi"("VRN IN"=w6130, "Bool Refnum"=w6107, "Commande #"=6, "Args"=w6105) -> ("VRN OUT"=w6108:refnum<visa-resource-name>, "Error OUT"=w6106:errorcluster)  [unwired: 9 in, 1 out]
                            n2320 = local write "TCS Error"(w6106) -> ()
                            n2321 = local write "TCS VRN"(w6108) -> ()
                            n2322 = local write "NO epoch"(w6113) -> ()
                            n2323 = local write "NO AM"(w6111) -> ()
                            n2324 = local write "NO HA"(w6112) -> ()
                            n2325 = local write "N.O. Déc."(w6114) -> ()
                            n2326 = local write "N.O. A.D."(w6115) -> ()
                          }
                          frame #1 {
                            n2327 = Index Array(array=w6140, index #1=5 ("index"), index #2=6 ("index")) -> (element #1=w6136:string, element #2=w6137:string)
                            n2328 = Not Equal?(x=w6137, y="") -> (x != y?=w6133:bool)
                            n2329 = Not Equal?(x="", y=w6136) -> (x != y?=w6134:bool)
                            n2330 = And(x=w6134, y=w6133) -> (x .and. y?=w6132:bool)
                            n2331 = case shown="True" w6132 {
                              selector: w6132 -> [w6142 _]
                              tunnel: [w6142 w6143] -> w6131
                              frame False {
                              }
                              frame True {
                                n2332 = Two Button Dialog(message="Désirez-vous également charger\nles paramètres de guidage ?  ", 1:"NON" ("F button name (\"Cancel\")"), 2:"OUI" ("T button name (\"OK\")")) -> (T button?=w6143:bool)
                              }
                            }
                          }
                          frame #2 {
                            # "Vérifier le fonctionnement réel de cette fonction ..."
                            n2333 = case shown="True" w6147 {
                              tunnel: w6148 -> [_ w6169]
                              frame False {
                              }
                              frame True {
                                w6160 = 60.0 ("x")
                                n2334 = call "Time-str-array-to-time-dbl-array.vi"("Array-str"=w6169) -> ("Array-dbl"=w6170:dbl[])
                                n2335 = Index Array(array=w6170, index #1=5, index #2=6, index #3=0 ("index"), index #4=1 ("index"), index #5=7 ("index"), index #6=8 ("index")) -> (element #1=w6173:dbl, element #2=w6171:dbl, element #3=w6172:dbl, element #4=w6150:dbl, element #5=w6166:dbl, element #6=w6165:dbl)
                                n2336 = Subtract(x=w6173, y=w6172) -> (x-y=w6161:dbl)
                                n2337 = Subtract(x=w6171, y=w6150) -> (x-y=w6162:dbl)
                                n2338 = Divide(x=w6150, y=180.0) -> (x/y=w6152:dbl)
                                n2339 = To Single Precision Float(number=w6166) -> (single precision float=w6163:sgl)
                                n2340 = To Single Precision Float(number=w6165) -> (single precision float=w6164:sgl)
                                n2341 = Multiply(x=w6160, y=w6161) -> (x*y=w6158:dbl)
                                n2342 = Multiply(x=w6160, y=w6162) -> (x*y=w6159:dbl)
                                n2343 = Multiply(x=3.141592653589793, y=w6152) -> (x*y=w6151:dbl)
